vi "input.vi"(10 "cutIndex":i32, 11 "file path":path) -> (0 "fs":dbl, 1 "ECG 2":dbl[](array[numeric]), 2 "ECG 1":dbl[](array[numeric]), 3 "Time":dbl[](array[numeric]), 4 "size(s)":i32, 6 "deltaTime":dbl[](array[numeric]))   [LabVIEW 2025]
uses:
  <vilib>/Analysis/baseanly.llb/Mean (DBL).vi
  <vilib>/Utility/file.llb/Read Delimited Spreadsheet (DBL).vi
  <vilib>/Analysis/NI_AALBase.lvlib
panel:
  out "mean":dbl format="%0.2f"
  out "Waveform Graph":dbl[](graph)
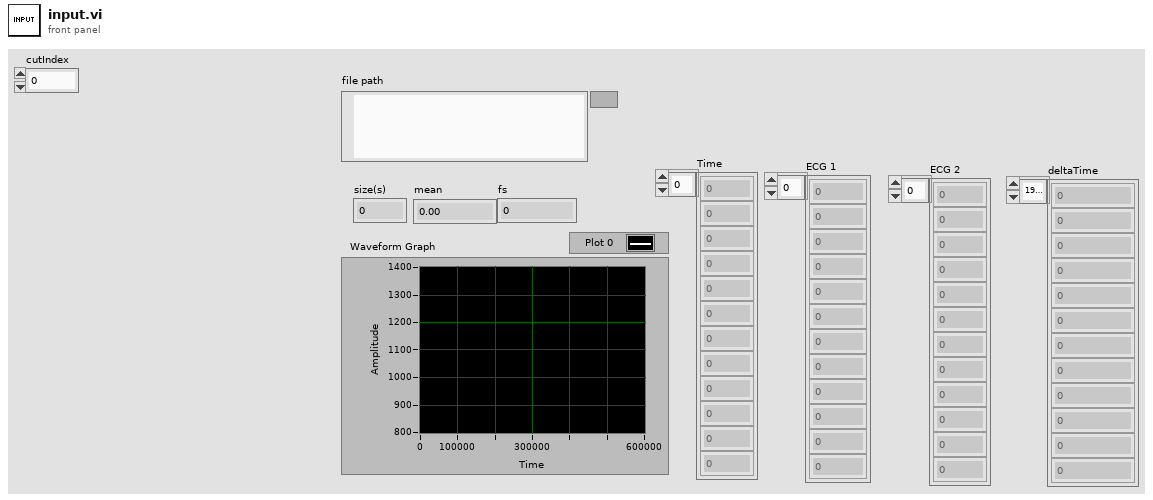
[diagram p1: front panel]
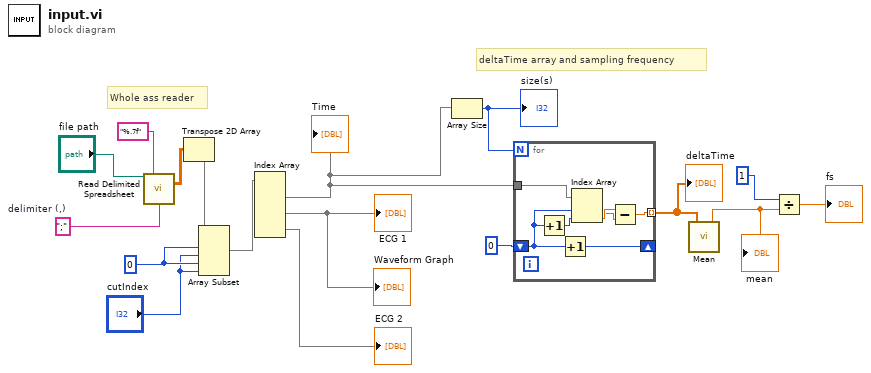
[diagram p0: block diagram]
diagram:
  w8 = 0
  w16 = ";"  # delimiter (,)
  # "deltaTime array and sampling frequency"
  # "Whole ass reader"
  n1 = call-poly <vilib>:"Read Delimited Spreadsheet.vi"("file path (dialog if empty)"="file path", "format (%.3f)"="%.7f", "delimiter (\\t)"=w16) -> ("all rows"=w13:dbl[][])  [unwired: 7 in, 5 out]
  n2 = Transpose 2D Array(2D array=w13) -> (transposed array=w10:dbl[][])
  n3 = Array Subset(array=w10, index (row)=w8, length (row)="cutIndex", index (col)=w8, length (col)="cutIndex") -> (w9:dbl[][])
  n4 = Index Array(array=w9) -> (element #1=w3:dbl[], element #2=→"ECG 1" →"Waveform Graph":dbl[], element #3=→"ECG 2":dbl[])  [unwired: 6 in]
  "Time" <- w3
  n5 = Array Size(array=w3) -> (size(s)=w12:i32)
  "size(s)" <- w12
  n6 = for {
    N: w12 -> [_]
    tunnel: w3 -> [w24]
    tunnel: [w22] -> w7 mode=indexing
    shift-right: [w18] -> _
    shift-left: 0 -> [w19]
    n7 = Increment(x=w19) -> (x+1=w23:i32)
    n8 = Increment(x=w19) -> (x+1=w18:i32)
    n9 = Index Array(array=w24, index #1=w19, index #2=w23) -> (element #1=w20:dbl, element #2=w21:dbl)
    n10 = Subtract(x=w21, y=w20) -> (x-y=w22:dbl)
  }
  "deltaTime" <- w7
  n11 = call-poly <vilib>:"Mean.vi"("X"=w7) -> ("mean"=w5:dbl)  [unwired: 1 out]
  "mean" <- w5
  n12 = Divide(x=1, y=w5) -> (x/y=→"fs":dbl)
